vi "FL Get Membership Function (MF Array).vi"(0 "membership functions in":T1[](array[typedef]) {"shape" items=["Triangle", "Trapezoid", "Singleton", "Sigmoid", "Gaussian", "User-Defined"]}, 3 "membership function index":i32, 11 "error in (no error)":errorcluster) -> (4 "membership functions out":T1[](array[typedef]) {"shape" items=["Triangle", "Trapezoid", "Singleton", "Sigmoid", "Gaussian", "User-Defined"]}, 6 "name":string, 8 "shape":T2 items=["Triangle", "Trapezoid", "Singleton", "Sigmoid", "Gaussian", "User-Defined"], 10 "points":dbl[](array[numeric]), 13 "user-defined shape index":i32, 14 "color":u32(colorbox), 15 "error out":errorcluster)   [LabVIEW 2013, in "NI_Fuzzy_Logic_API.lvlib"]
doc: "Returns the shape, color, and points of a membership function for a linguistic variable. You can return a membership function from a fuzzy system or from an array of membership functions. The data type you wire to the <B>fuzzy system in</B> input determines the polymorphic instance to use."
uses:
  <vilib>/addons/Fuzzy Logic/NI_Fuzzy_Logic_API.lvlib
  <vilib>/addons/Fuzzy Logic/TypeDefs/FL Membership Function Shape.ctl
  <vilib>/addons/Fuzzy Logic/TypeDefs/FL Membership Function.ctl
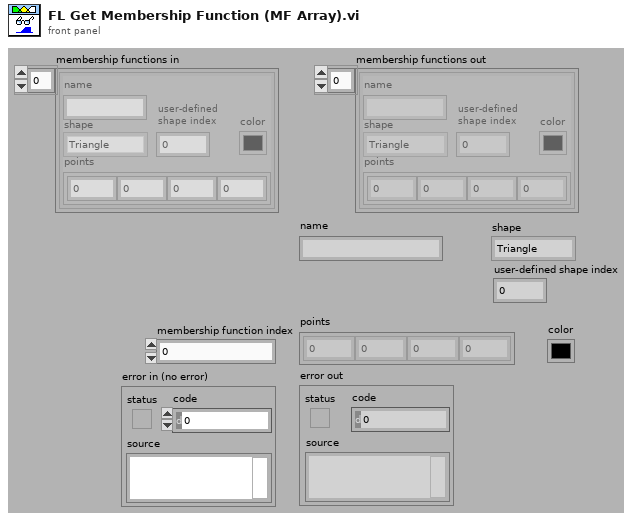
[diagram p1: front panel]
types:
  T1 = typedef "NI_Fuzzy_Logic_API.lvlib/FL Membership Function.ctl" = cluster{"name":string, "shape":T2, "points":dbl[], "color":u32, "user-defined shape index":i32}
  T2 = typedef "NI_Fuzzy_Logic_API.lvlib/FL Membership Function Shape.ctl" = u16
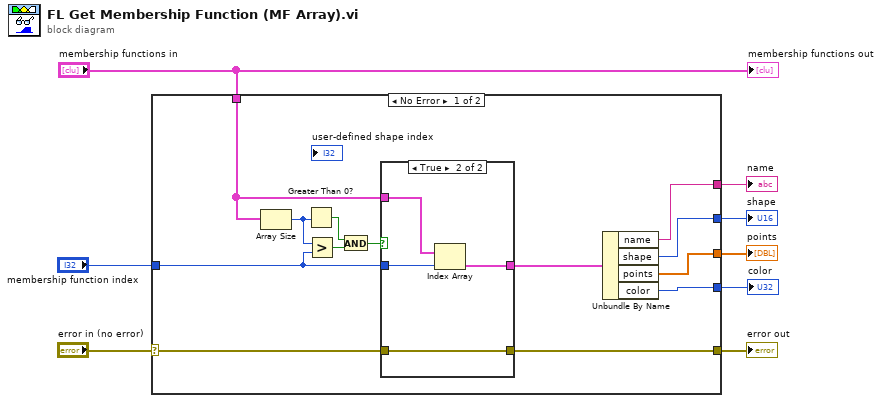
[diagram p0: block diagram]
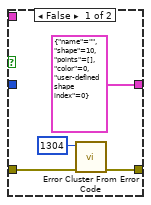
[diagram p2: hidden frame]
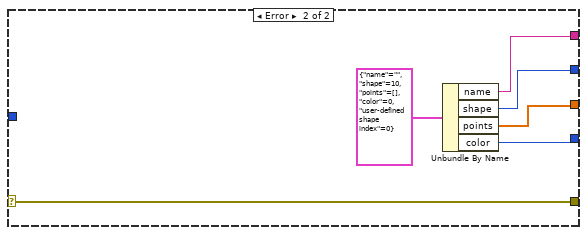
[diagram p3: hidden frame]
diagram:
  n1 = case shown="No Error" "error in (no error)" {
    selector: "error in (no error)" -> [w11 w35]
    tunnel: "membership function index" -> [w12 _]
    tunnel: [w20 w34] -> w7
    tunnel: [w18 w32] -> w6
    tunnel: [w17 w31] -> w5
    tunnel: [w19 w33] -> w4
    tunnel: [w10 w35] -> w2
    tunnel: "membership functions in" -> [w13 _]
    frame No Error {
      n2 = Array Size(array=w13) -> (size(s)=w15:i32)
      n3 = Greater Than 0?(x=w15) -> (x > 0?=w14:bool)
      n4 = Greater?(x=w15, y=w12) -> (0:w16:bool)
      n5 = And(x=w14, y=w16) -> (x .and. y?=w9:bool)
      n6 = case shown="True" w9 {
        tunnel: [T1 {"name"="", "shape"=10, "points"=[], "color"=0, "user-defined shape index"=0} ("MF") w29] -> w21
        tunnel: w13 -> [_ w28]
        tunnel: w12 -> [_ w27]
        tunnel: w11 -> [w24 w26]
        tunnel: [w23 w26] -> w10
        frame False {
          n7 = call <vilib>:"Error Cluster From Error Code.vi"("error in (no error)"=w24, "error code (0)"=1304) -> ("error out"=w23:errorcluster)  [unwired: 1 in, 6 out]
        }
        frame True {
          n8 = Index Array(array=w28, index=w27) -> (element=w29:T1)
        }
      }
      n9 = Unbundle By Name(w21) -> ("name"=w20:string, "shape"=w19:T2, "points"=w18:dbl[], "color"=w17:u32)
    }
    frame Error {
      n10 = Unbundle By Name(T1 {"name"="", "shape"=10, "points"=[], "color"=0, "user-defined shape index"=0} ("MF")) -> ("name"=w34:string, "shape"=w33:T2, "points"=w32:dbl[], "color"=w31:u32)
    }
  }
  "name" <- w7
  "points" <- w6
  "color" <- w5
  "shape" <- w4
  "error out" <- w2
  "membership functions out" <- "membership functions in"
